vi "getType.vi"(8 "error in (no error)":errorcluster, 11 "Decoration In":refnum<class "Terminal.lvclass">) -> (0 "error out":errorcluster, 2 "type":refnum<vi>, 3 "Decoration Out":refnum<class "Terminal.lvclass">)   [LabVIEW 2023, in "TLC_Scripto.lvlib" / "Terminal.lvclass"]
uses:
  Terminal.lvclass
  Terminal.lvclass/Terminal.ctl
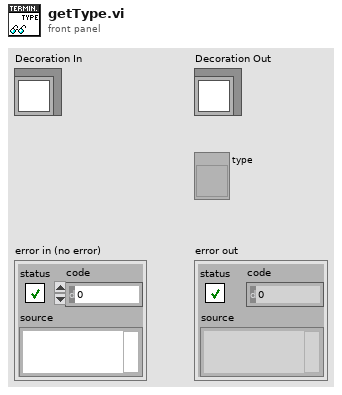
[diagram p1: front panel]
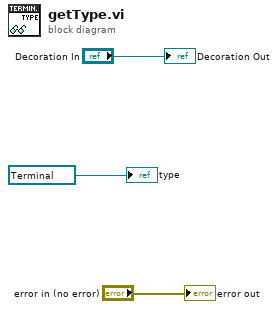
[diagram p0: block diagram]
diagram:
  "error out" <- "error in (no error)"
  "Decoration Out" <- "Decoration In"
  "type" <- refnum<vi> refnum ("type")
